vi "main3.vi"   [LabVIEW 2014]
uses:
  src/user.lib/_NEVSTOP/GlobalStop/_gStop.vi
  src/user.lib/_NEVSTOP/GlobalStop/GSTOP.lvlib
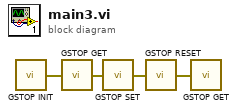
[diagram p0: block diagram]
diagram:
  n1 = call "GSTOP INIT.vi"() -> ("error out"=w4:errorcluster)  [unwired: 15 in]
  n2 = call "GSTOP GET.vi"("error in (no error)"=w4) -> ("error out"=w3:errorcluster)  [unwired: 13 in, 1 out]
  n3 = call "GSTOP SET.vi"("error in (no error)"=w3) -> ("error out"=w2:errorcluster)  [unwired: 14 in]
  n4 = call "GSTOP RESET.vi"("error in (no error)"=w2) -> ("error out"=w1:errorcluster)  [unwired: 14 in]
  n5 = call "GSTOP GET.vi"("error in (no error)"=w1) -> ()  [unwired: 13 in, 2 out]
